vi "Error_Query.vi"(8 "error in (no error)":errorcluster, 11 "VISA resource name":refnum<visa-resource-name>) -> (0 "error out":errorcluster, 1 "Error Message":string, 2 "Error Code":i32[](array[numeric]), 3 "VISA resource name out":refnum<visa-resource-name>)   [LabVIEW 2011]
doc: "Queries an instrument for any errors in the error queue of the instrument. The tkdpo4k Error Query VI continuously reads errors until this VI reads all the errors from the instrument. \n<B>Note</B>: Because most driver VIs automatically call the tkdpo4k Error Query VI, you do not need to call this VI in an application."
uses:
  <instrlib>/Tektronix 7000 Series/Tektronix 7000 Series.lvlib
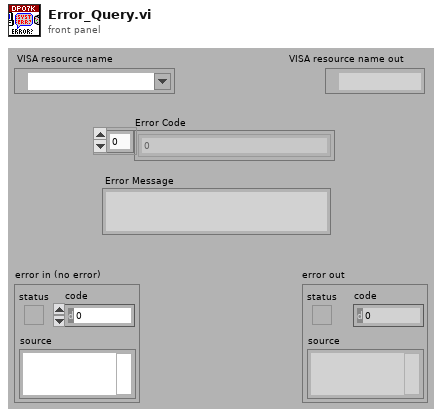
[diagram p1: front panel]
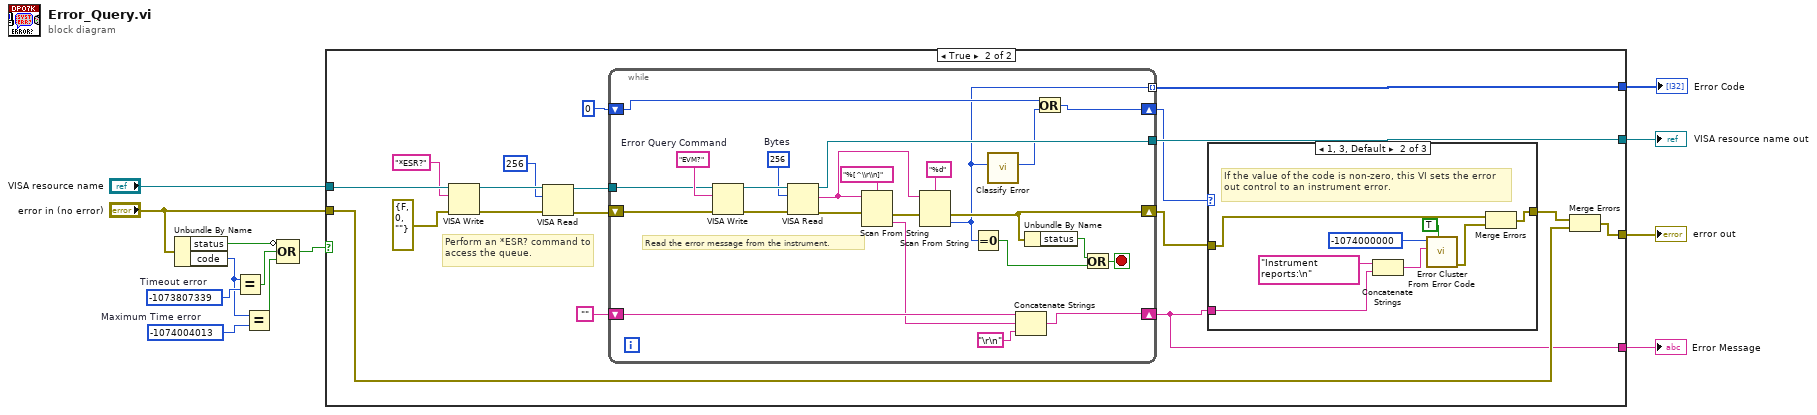
[diagram p0: block diagram]
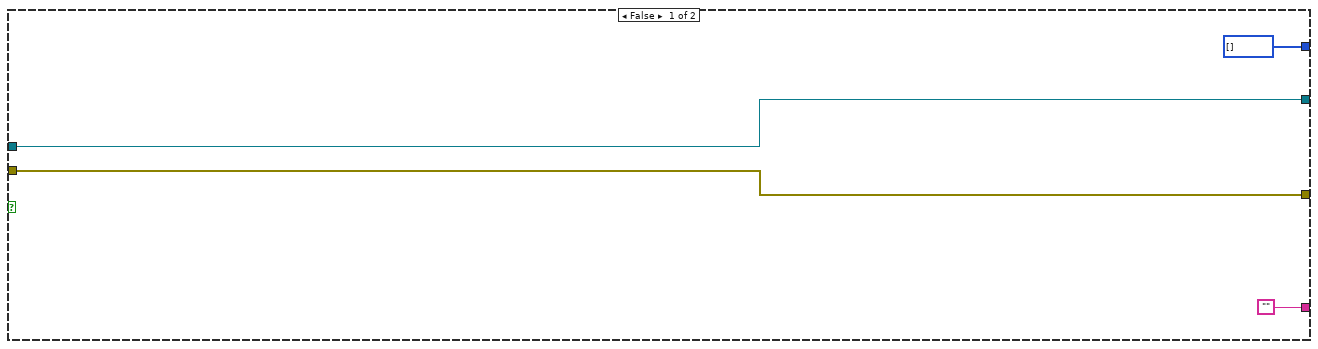
[diagram p2: hidden frame]
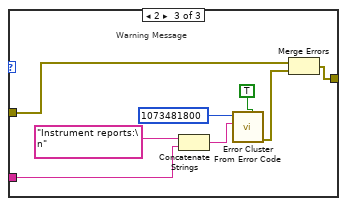
[diagram p4: hidden frame]
diagram:
  w3 = -1074004013  # Maximum Time error
  w8 = -1073807339  # Timeout error
  n1 = Unbundle By Name("error in (no error)") -> ("status"=w9:bool, "code"=w2:i32)
  n2 = Equal?(x=w2, y=w8) -> (x = y?=w7:bool)
  n3 = Equal?(x=w2, y=w3) -> (x = y?=w1:bool)
  n4 = Compound Arithmetic op=OR(invert w9, w7, w1) -> (w6:bool)
  n5 = case shown="True" w6 {
    tunnel: [w17 w35] -> w13
    tunnel: "VISA resource name" -> [w17 w30]
    tunnel: "error in (no error)" -> [w16 w24]
    tunnel: [w16 w33] -> w11
    tunnel: ["" w18] -> w5
    tunnel: [i32[] [] w31] -> w4
    frame False {
    }
    frame True {
      # "Perform an *ESR? command to access the queue."
      n6 = VISA Write(VISA resource name=w30, write buffer="*ESR?", error in (no error)=errorcluster {"status"=FALSE, "code"=0, "source"=""}) -> (VISA resource name out=w27:refnum<visa-resource-name>, error out=w28:errorcluster)  [unwired: 1 out]
      n7 = VISA Read(VISA resource name=w27, byte count=u32 256, error in (no error)=w28) -> (VISA resource name out=w25:refnum<visa-resource-name>, error out=w23:errorcluster)  [unwired: 2 out]
      n8 = while {
        tunnel: [w76] -> w35
        tunnel: w25 -> [w59]
        shift-right: [w65] -> w18
        shift-left: "" -> [w67]
        shift-right: [w55] -> w20
        shift-left: 0 -> [w56]
        shift-right: [w63] -> w21
        shift-left: w23 -> [w64]
        tunnel: [w53] -> w31 mode=indexing
        stop <- w70 stop-if-true
        w74 = u32 256  # Bytes
        w72 = "EVM?"  # Error Query Command
        # "Read the error message from the instrument."
        n9 = VISA Write(VISA resource name=w59, write buffer=w72, error in (no error)=w64) -> (VISA resource name out=w75:refnum<visa-resource-name>, error out=w73:errorcluster)  [unwired: 1 out]
        n10 = VISA Read(VISA resource name=w75, byte count=w74, error in (no error)=w73) -> (VISA resource name out=w76:refnum<visa-resource-name>, read buffer=w68:string, error out=w62:errorcluster)  [unwired: 1 out]
        n11 = Scan From String(format string="%[^\\r\\n]", input string=w68, error in=w62) -> (error out=w61:errorcluster, output 1=w66:string)  [unwired: 2 in, 2 out]
        n12 = Scan From String(format string="%d", input string=w68, error in=w61) -> (error out=w63:errorcluster, output 1=w53:i32)  [unwired: 2 in, 2 out]
        n13 = Equal To 0?(x=w53) -> (x = 0?=w58:bool)
        n14 = call <instrlib>:"Classify Error.vi"("Error Code"=w53) -> ("Error Classification"=w54:u32)  [unwired: 10 in]
        n15 = Concatenate Strings(w67, w66, "\r\n") -> (w65:string)
        n16 = Unbundle By Name(w63) -> ("status"=w60:bool)
        n17 = Or(x=w56, y=w54) -> (x .or. y?=w55:u32)
        n18 = Or(x=w60, y=w58) -> (x .or. y?=w70:bool)
      }
      n19 = case shown="1, 3, Default" w20 {
        tunnel: [w36 w37 w45] -> w19
        tunnel: w18 -> [_ w40 w49]
        tunnel: w21 -> [w36 w39 w47]
        frame 0 {
        }
        frame 1, 3, Default {
          # "If the value of the code is non-zero, this VI sets the error out control to an instrument error."
          n20 = Concatenate Strings("Instrument reports:\n" ("Source"), w40) -> (w41:string)
          n21 = call <vilib>:"Error Cluster From Error Code.vi"("show call chain? (False)"=TRUE, "error message (\"\")"=w41, "error code (0)"=-1074000000 ("Code")) -> ("error out"=w38:errorcluster)  [unwired: 6 in]
          n22 = Merge Errors(w39, w38) -> (w37:errorcluster)
        }
        frame 2 {
          # "Warning Message"
          n23 = Concatenate Strings("Instrument reports:\n" ("Source"), w49) -> (w50:string)
          n24 = call <vilib>:"Error Cluster From Error Code.vi"("is warning? (False)"=TRUE ("show call chain? (False)"), "error message (\"\")"=w50, "error code (0)"=1073481800 ("Code")) -> ("error out"=w46:errorcluster)  [unwired: 6 in]
          n25 = Merge Errors(w47, w46) -> (w45:errorcluster)
        }
      }
      n26 = Merge Errors(w19, w24) -> (w33:errorcluster)
    }
  }
  "VISA resource name out" <- w13
  "error out" <- w11
  "Error Message" <- w5
  "Error Code" <- w4
